vi "Close UI.vi"(8 "error in (no error)":errorcluster, 11 "Actor wUI in":refnum<class "Actor wUI.lvclass">) -> (0 "error out":errorcluster, 3 "Actor wUI out":refnum<class "Actor wUI.lvclass">)   [LabVIEW 2017, in "Framework.lvlib" / "Actor wUI.lvclass"]
uses:
  Actor wUI.lvclass
  Actor wUI.lvclass/Actor wUI.ctl
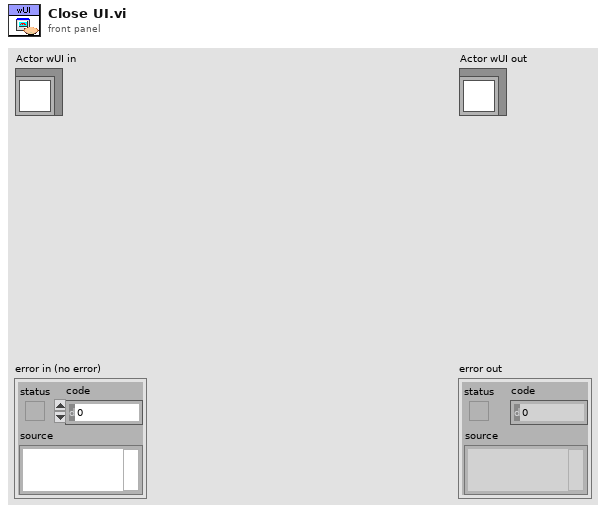
[diagram p1: front panel]
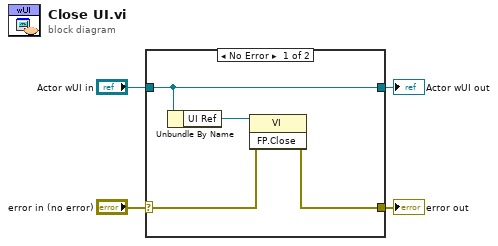
[diagram p0: block diagram]
diagram:
  n1 = case shown="No Error" "error in (no error)" {
    selector: "error in (no error)" -> [w6 w10]
    tunnel: [w5 w10] -> w3
    tunnel: [w8 w9] -> w1
    tunnel: "Actor wUI in" -> [w8 w9]
    frame No Error {
      n2 = Unbundle By Name(w8) -> ("UI Ref"=w7:refnum<vi>)
      n3 = invoke class="VI" method="FP.Close"(reference=w7, error in=w6) -> (error out=w5:errorcluster)  [unwired: 1 in, 2 out]
    }
    frame Error {
    }
  }
  "error out" <- w3
  "Actor wUI out" <- w1
